vi "Set Temperature Set Point.vi"(8 "error in (no error)":errorcluster, 11 "Temperature Set Point (deg C)":dbl) -> (0 "error out":errorcluster)   [LabVIEW 2015, in "Thermal Chamber Response Simulator.lvlib"]
doc: "Assign set point in simulator AE.\n____\nDelacor QMH Thermal Chamber Examples 4.0.0.21\nCopyright (c) 2018, Delacor"
uses:
  Thermal Chamber Response Simulator.lvlib
  Action--enum.ctl
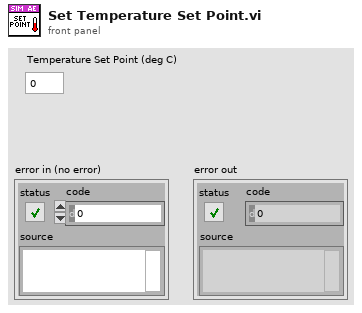
[diagram p1: front panel]
types:
  T1 = typedef "Thermal Chamber Response Simulator.lvlib/Action--enum.ctl" = enum16{"Initialize", "Set Temperature Required", "Set Ramp Rate", "Get Status", "Disable Heater", "Enable Heater", "Exit Application"}
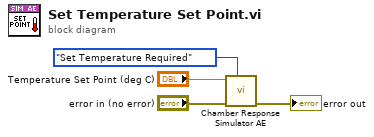
[diagram p0: block diagram]
diagram:
  n1 = call "Chamber Response Simulator AE.vi"("Thermal Chamber Function"=Action--enum."Set Temperature Required", "error in (no error)"="error in (no error)", "Temperature Set Point in"="Temperature Set Point (deg C)") -> ("error out"=→"error out":errorcluster)  [unwired: 3 in, 5 out]
